vi "CalculateCustomBlinkTransitions.vi"(11 "custom blink":T2) -> (3 "custom blink internal state":T1)   [LabVIEW 2017, in "BlinkProcess.lvlib"]
uses:
  <vilib>/addons/BlinkProcess/BlinkProcess.lvlib
  <vilib>/addons/BlinkProcess/controls/customBlinkConfig.ctl
  <vilib>/addons/BlinkProcess/controls/CustomBlinkInternalState.ctl
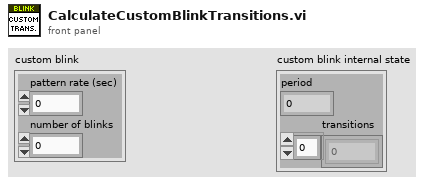
[diagram p1: front panel]
types:
  T1 = typedef "BlinkProcess.lvlib/CustomBlinkInternalState.ctl" = cluster{"period":i32, "transitions":i32[]}
  T2 = typedef "BlinkProcess.lvlib/customBlinkConfig.ctl" = cluster{"pattern rate (sec)":dbl, "number of blinks":u32}
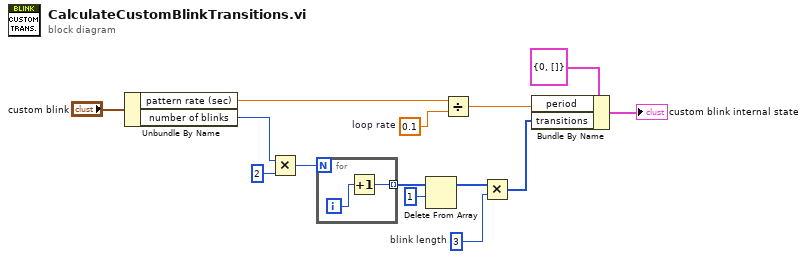
[diagram p0: block diagram]
diagram:
  w5 = 3  # blink length
  w11 = 0.1  # loop rate
  n1 = Unbundle By Name("custom blink") -> ("pattern rate (sec)"=w12:dbl, "number of blinks"=w3:u32)
  n2 = Multiply(x=w3, y=2) -> (x*y=w2:u32)
  n3 = for {
    N: w2 -> [_]
    tunnel: [w15] -> w8 mode=indexing
    i -> [w16]
    n4 = Increment(x=w16) -> (x+1=w15:i32)
  }
  n5 = Delete From Array(array=w8, length=1) -> (array with subset deleted=w6:i32[])  [unwired: 1 in, 1 out]
  n6 = Divide(x=w12, y=w11) -> (x/y=w10:dbl)
  n7 = Multiply(x=w6, y=w5) -> (x*y=w4:i32[])
  n8 = Bundle By Name(cluster=T1 {"period"=0, "transitions"=[]} ("customBlinkInternalState"), "period"=w10, "transitions"=w4) -> (→"custom blink internal state":T1)
